vi "UtilityLib.set color of listbox.vi"(0 "listboxRef":refnum<vi>, 2 "valueStatus":T1, 5 "error in (no error)":errorcluster) -> (19 "error out":errorcluster)   [LabVIEW 2015, in "UtilityLib.lvlib"]
doc: "Changes the color of a listbox to values defined in six-color vi."
uses:
  UtilityLib.lvlib
  UtilityLib.valueStatus.ctl
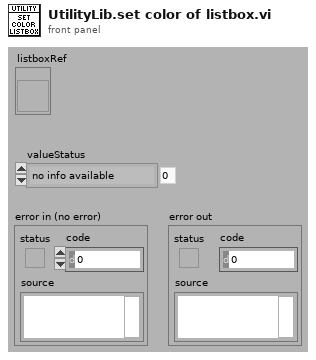
[diagram p1: front panel]
types:
  T1 = typedef "UtilityLib.lvlib/UtilityLib.valueStatus.ctl" = enum16{"no info available", "stand by/off", "on", "warning", "alarm/malfunction", "not implemented", "user action required", "important information", "system default", "control default", "indicator default", "button default"}
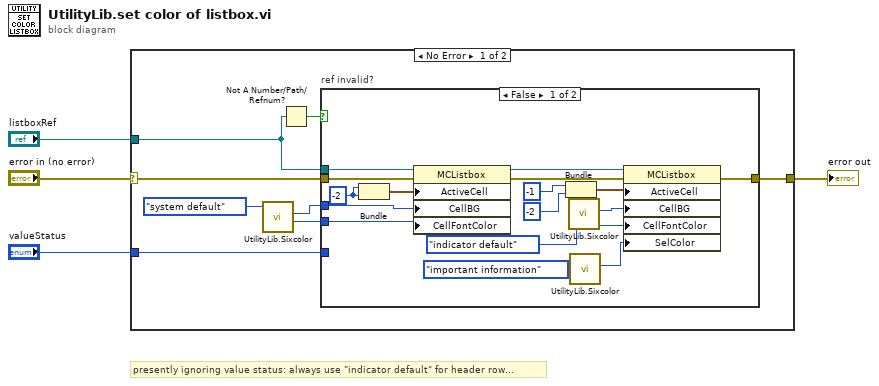
[diagram p0: block diagram]
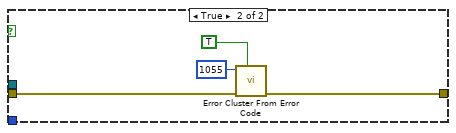
[diagram p2: hidden frame]
diagram:
  # "presently ignoring value status: always use \"indicator default\" for header row..."
  n1 = case shown="No Error" "error in (no error)" {
    selector: "error in (no error)" -> [w5 w34]
    tunnel: [w12 w34] -> w4
    tunnel: "listboxRef" -> [w8 _]
    tunnel: "valueStatus" -> [w6 _]
    frame No Error {
      n2 = call "UtilityLib.Sixcolor.vi"("State"=UtilityLib.valueStatus."system default") -> ("elementBackground"=w11:u32, "elementText"=w10:u32)  [unwired: 2 in, 2 out]
      n3 = Not A Number/Path/Refnum?(number/path/refnum=w8) -> (NaN/Path/Refnum?=w9:bool)
      n4 = case "ref invalid?" shown="False" w9 {
        tunnel: [w21 w32] -> w12
        tunnel: w5 -> [w29 w33]
        tunnel: w8 -> [w28 _]
        tunnel: w11 -> [w25 _]
        tunnel: w10 -> [w24 _]
        tunnel: w6 -> [_ _]
        frame False {
          w26 = -2
          n5 = Bundle(w26, w26) -> (w27:cluster{i32, i32})  [unwired: 1 in]
          n6 = property class="MCListbox"(reference=w28, error in=w29, "ActiveCell"=w27, "CellBG"=w25, "CellFontColor"=w24) -> (reference out=w23:refnum<vi>, error out=w22:errorcluster)
          n7 = Bundle(-1, -2) -> (w18:cluster{i32, i32})  [unwired: 1 in]
          n8 = call "UtilityLib.Sixcolor.vi"("State"=UtilityLib.valueStatus."indicator default") -> ("elementBackground"=w17:u32, "elementText"=w16:u32)  [unwired: 2 in, 2 out]
          n9 = call "UtilityLib.Sixcolor.vi"("State"=UtilityLib.valueStatus."important information") -> ("elementBackground"=w14:u32)  [unwired: 2 in, 3 out]
          n10 = property class="MCListbox"(reference=w23, error in=w22, "ActiveCell"=w18, "CellBG"=w17, "CellFontColor"=w16, "SelColor"=w14) -> (error out=w21:errorcluster)  [unwired: 1 out]
        }
        frame True {
          n11 = call <vilib>:"Error Cluster From Error Code.vi"("show call chain? (False)"=TRUE, "error in (no error)"=w33, "error code (0)"=1055) -> ("error out"=w32:errorcluster)  [unwired: 6 in]
        }
      }
    }
    frame Error {
    }
  }
  "error out" <- w4
